vi "Path.vi"(8 "error in (no error)":errorcluster, 10 "pathname":string, 11 "Masterv2 in":refnum<class "Masterv2.lvclass">) -> (0 "error out":errorcluster, 3 "Masterv2 out":refnum<class "Masterv2.lvclass">)   [LabVIEW 2014, in "Main Libraryv2.lvlib" / "Masterv2.lvclass"]
uses:
  Master/Masterv2.lvclass
panel:
  out "appended path":path
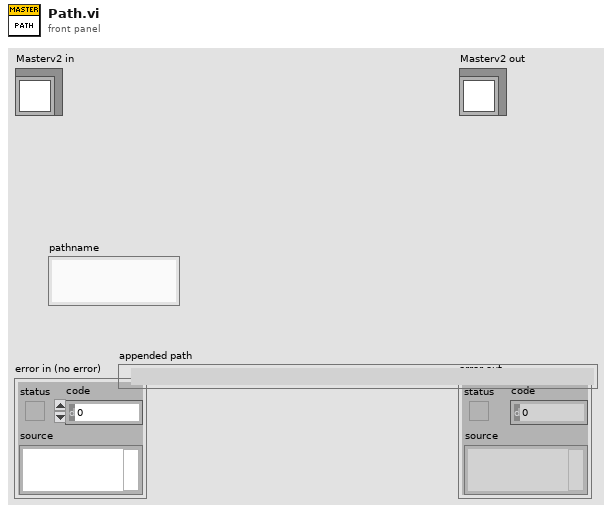
[diagram p1: front panel]
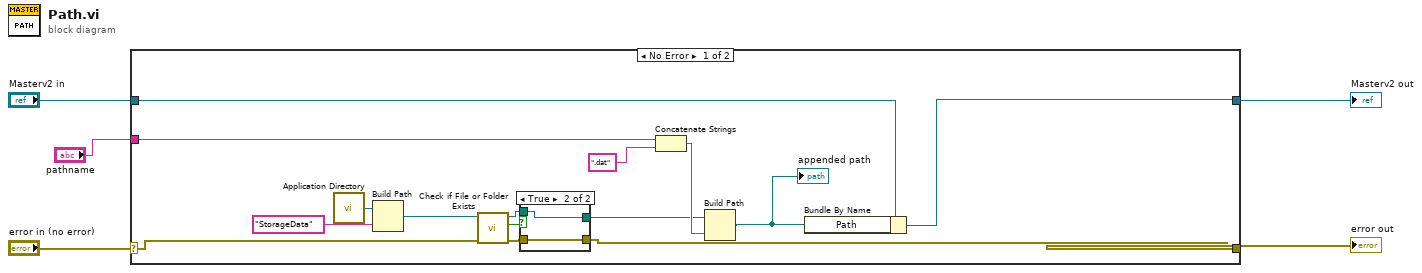
[diagram p0: block diagram]
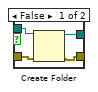
[diagram p2: hidden frame]
diagram:
  n1 = case shown="No Error" "error in (no error)" {
    selector: "error in (no error)" -> [w14 w28]
    tunnel: [w6 w28] -> w4
    tunnel: [w11 w27] -> w2
    tunnel: "Masterv2 in" -> [w12 w27]
    tunnel: "pathname" -> [w13 _]
    frame No Error {
      n2 = call <vilib>:"Application Directory.vi"() -> ("Application Directory"=w20:path)
      n3 = Build Path(base path=w20, name or relative path="StorageData") -> (appended path=w15:path)
      n4 = call <vilib>:"Check if File or Folder Exists.vi"("error in (no error)"=w14, "path"=w15) -> ("error out"=w8:errorcluster, "file or folder exists?"=w10:bool, "dup path"=w9:path)  [unwired: 7 in]
      n5 = case shown="True" w10 {
        tunnel: w9 -> [w24 w26]
        tunnel: w8 -> [w23 w25]
        tunnel: [w22 w26] -> w7
        tunnel: [w21 w25] -> w6
        frame False {
          n6 = Create Folder(path (use dialog)=w24, error in=w23) -> (created path=w22:path, error out=w21:errorcluster)  [unwired: 1 in, 1 out]
        }
        frame True {
        }
      }
      n7 = Concatenate Strings(w13, ".dat" ("string")) -> (w18:string)
      n8 = Build Path(base path=w7, name or relative path=w18) -> (appended path=w16:path)
      "appended path" <- w16
      n9 = Bundle By Name(cluster=w12, "Path"=w16) -> (w11:refnum<class "Masterv2.lvclass">)
    }
    frame Error {
    }
  }
  "error out" <- w4
  "Masterv2 out" <- w2
